vi "4.5.vi"() -> ()   [LabVIEW 2017]
panel:
  out "循坏执行的次数":dbl
  in  "指定值":dbl
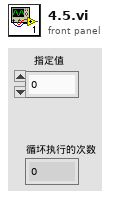
[diagram p1: front panel]
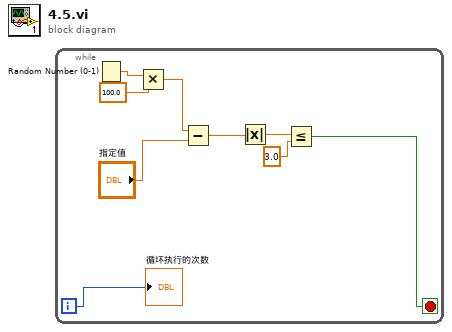
[diagram p0: block diagram]
diagram:
  n1 = while {
    i -> [w4]
    stop <- w1 stop-if-true
    n2 = Random Number (0-1)() -> (number: 0 to 1=w9:dbl)
    n3 = Multiply(x=w9, y=100.0) -> (x*y=w7:dbl)
    n4 = Subtract(x=w7, y="指定值") -> (x-y=w5:dbl)
    n5 = Absolute Value(x=w5) -> (abs(x)=w3:dbl)
    n6 = Less Or Equal?(x=w3, y=3.0) -> (x <= y?=w1:bool)
    "循坏执行的次数" <- w4
  }
